vi "Get Available Versions.vi"(11 "WebView2 Updater in":refnum<class "WebView2 Updater.lvclass">) -> (0 "error out":errorcluster, 3 "WebView2 Updater out":refnum<class "WebView2 Updater.lvclass">)   [LabVIEW 2020, in "WebView2 Updater.lvclass"]
uses:
  WebView2 Updater.lvclass
  WebView2 Updater.lvclass/WebView2 Updater.ctl
  <vilib>/httpClient/LabVIEWHTTPClient.lvlib
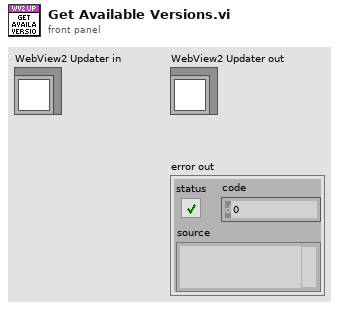
[diagram p1: front panel]
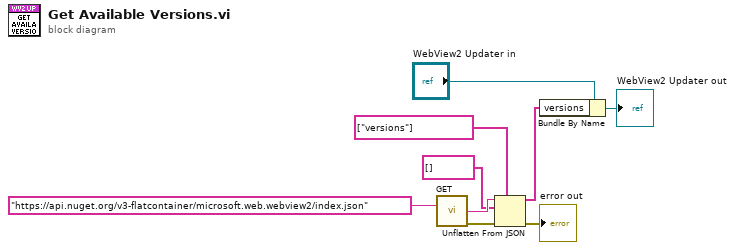
[diagram p0: block diagram]
diagram:
  n1 = call <vilib>:"GET.vi"("url"="https://api.nuget.org/v3-flatcontainer/microsoft.web.webview2/index.json") -> ("body"=w5:string, "error out"=w4:errorcluster)  [unwired: 11 in, 2 out]
  n2 = Unflatten From JSON(path=string[] ["versions"], JSON string=w5, type and defaults=string[] [] ("versions"), error in (no error)=w4) -> (value=w8:string[], error out=→"error out":errorcluster)  [unwired: 3 in]
  n3 = Bundle By Name(cluster="WebView2 Updater in", "versions"=w8) -> (→"WebView2 Updater out":refnum<class "WebView2 Updater.lvclass">)
